vi "DronePi Main.vi"() -> ()   [LabVIEW 2014]
uses:
  SubVI/Aircraft Information/Controls/Drone Information.ctl
  SubVI/Aircraft Information/Controls/Base Mode.ctl
  SubVI/Aircraft Information/Controls/Aircraft Mode.ctl
  SubVI/Aircraft Information/Controls/Aircraft Sensor Status Data.ctl
  SubVI/GUI Design/Indicators/Sensor Status LED CLuster.ctl
  SubVI/GUI Design/Indicators/Status LED.ctl
  SubVI/Aircraft Information/Controls/Aircraft GPS Data.ctl
  SubVI/Aircraft Information/Controls/GPS Fix Type.ctl
  SubVI/Aircraft Information/Controls/Aircraft Attitude Data.ctl
  <vilib>/Platform/TimedLoop/XDataNode/timing_clust.ctl
  <vilib>/Platform/TimedLoop/XDataNode/nitl_modes.ctl
  <vilib>/Platform/TimedLoop/XDataNode/wakeup.ctl
  SubVI/Aircraft Information/Sub VI/Selected Aircraft/SubVI/Set Selected Aircraft.vi
  Web Services/DronePi Global Variables.vi
  SubVI/Aircraft Information/Sub VI/Selected Aircraft/SubVI/Get Selected Aircraft.vi
  SubVI/Aircraft Information/Sub VI/Get Aircraft Attitude.vi
  SubVI/Aircraft Information/Sub VI/Get Aircraft GPS.vi
  SubVI/Aircraft Information/Sub VI/Get Aircraft System Status.vi
  SubVI/Aircraft Information/Sub VI/Get Aircraft Information.vi
  <vilib>/platform/TimedLoop/XDataNode/XDataNode.xnode
  <vilib>/Platform/TimedLoop/XDataNode/XDNodeRunTimeDep.lvlib
panel:
  out "Aircraft Att Data Out":T1
  out "Aircraft GPS Data Out":T2
  out "System Status Out":T4 {"Communication Drop Rate (%)" scale=0.0..100.0; "Battery Remaining (%)" scale=0.0..100.0; "CPU Load (%)" scale=0.0..100.0}
  out "Aircraft Information Out":T7={"Aircraft ID"=0, "Tag ID"="", "System Status"="", "Base Mode"={"Custom Mode"=FALSE, "Test Enabled"=FALSE, "Autonomous Mode"=FALSE, "Guided Mode"=FALSE, "Stabilization Enabled"=FALSE, "HIL Enabled"=FALSE, "Manual Mode"=FALSE, "Arm"=FALSE}, "Armed/Disarmed"=FALSE, "Battery Voltage"=0.0, "Control Mode"=enum."Stabalise", "Initialisation"=0, "Coms with aircraft good"=FALSE, "Mode"="", "Mission Uploaded"=FALSE} {"Initialisation" scale=0.0..100.0}
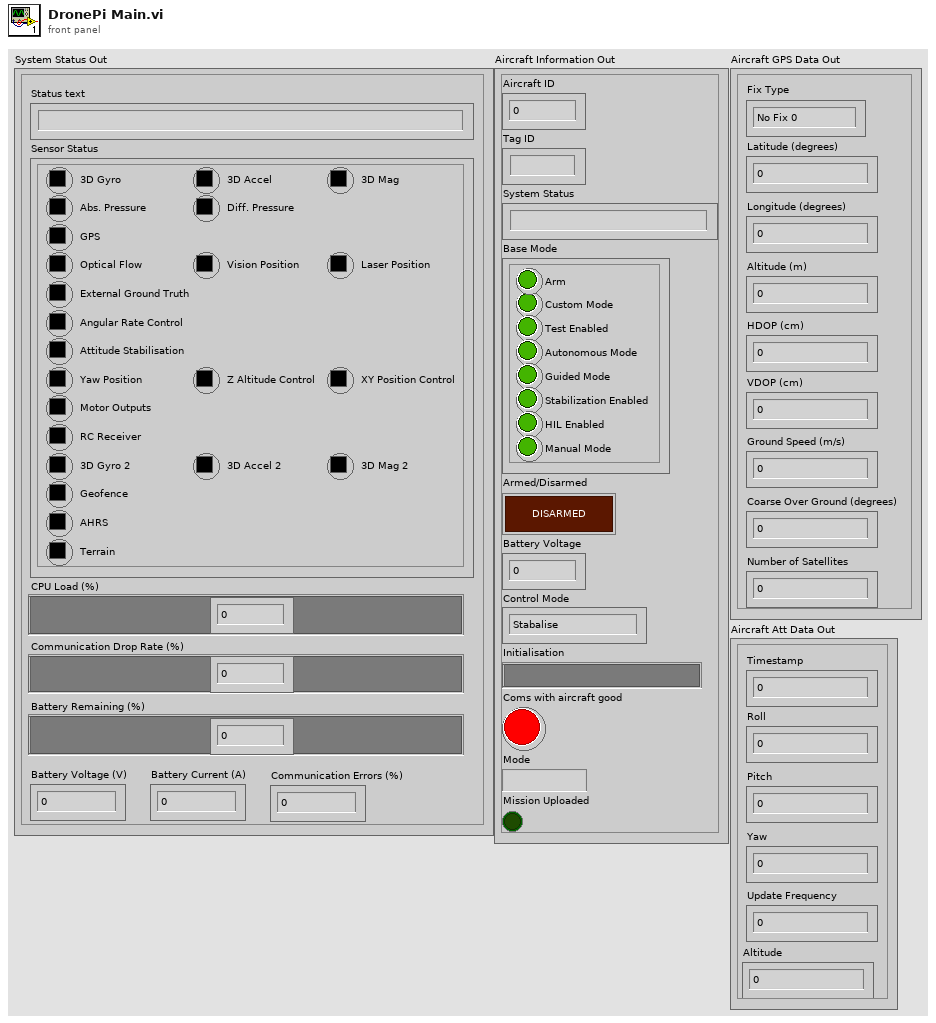
[diagram p1: front panel]
types:
  T1 = typedef "Aircraft Attitude Data.ctl" = cluster{"Roll":sgl, "Pitch":sgl, "Yaw":sgl, "Timestamp":u32, "Update Frequency":dbl, "Altitude":sgl}
  T2 = typedef "Aircraft GPS Data.ctl" = cluster{"Latitude (degrees)":dbl, "Longitude (degrees)":dbl, "Altitude (m)":dbl, "Fix Type":T3, "HDOP (cm)":u16, "VDOP (cm)":u16, "Ground Speed (m/s)":dbl, "Coarse Over Ground (degrees)":u16, "Number of Satellites":u8}
  T3 = typedef "GPS Fix Type.ctl" = enum16{"No Fix 0", "No Fix 1", "2D Fix", "3D Fix", "DGPS", "RTK"}
  T4 = typedef "Aircraft Sensor Status Data.ctl" = cluster{"Sensor Status":T5, "CPU Load (%)":dbl, "Battery Voltage (V)":dbl, "Battery Current (A)":dbl, "Battery Remaining (%)":dbl, "Communication Drop Rate (%)":dbl, "Communication Errors (%)":dbl, "Status text":string}
  T5 = typedef "Sensor Status LED CLuster.ctl" = cluster{"3D Gyro":u32, "3D Accel":u32, "3D Mag":u32, "Abs. Pressure":u32, "Diff. Pressure":u32, "GPS":T6, "Optical Flow":u32, "Vision Position":u32, "Laser Position":u32, "External Ground Truth":u32, "Angular Rate Control":u32, "Attitude Stabilisation":u32, "Yaw Position":u32, "Z Altitude Control":u32, "XY Position Control":u32, "Motor Outputs":u32, "RC Receiver":u32, "3D Gyro 2":u32, "3D Accel 2":u32, "3D Mag 2":u32, "Geofence":u32, "AHRS":u32, "Terrain":u32}
  T6 = typedef "Status LED.ctl" = u32
  T7 = typedef "Drone Information.ctl" = cluster{"Aircraft ID":u8, "Tag ID":string, "System Status":string, "Base Mode":T8, "Armed/Disarmed":bool, "Battery Voltage":dbl, "Control Mode":T9, "Initialisation":u8, "Coms with aircraft good":bool, "Mode":string, "Mission Uploaded":bool}
  T8 = typedef "Base Mode.ctl" = cluster{"Custom Mode":bool, "Test Enabled":bool, "Autonomous Mode":bool, "Guided Mode":bool, "Stabilization Enabled":bool, "HIL Enabled":bool, "Manual Mode":bool, "Arm":bool}
  T9 = typedef "Aircraft Mode.ctl" = enum16{"Loiter", "Stabalise", "Failsafe", "Emergency Stop"}
  T10 = typedef "XDNodeRunTimeDep.lvlib/timing_clust.ctl" = cluster{"Expected End [f-1]":u64, "Actual End [f-1]":u64, "Finished Late? [f-1]":bool, "Expected End [i-1]":u64, "Actual End [i-1]":u64, "Finished Late? [i-1]":bool, "Expected Start [i]":u64, "Actual Start [i]":u64, "Expected Start [f]":u64, "Actual Start [f]":u64, "Source Name":string, "Structure Name":string, "Period":i64, "Deadline":i64, "Offset":i64, "Start":i64, "Priority":i32, "Timeout":i32, "Mode":T11, "Wakeup Reason":T12, "Error":errorcluster, "Source Type":string, "Secondary Source Type":string, "Global End Time":u64, "Global Start Time":u64, "Frame Duration":u64, "Iteration Duration":u64, "Assigned CPU":i32, "I/O Scan Engine Mode":u32}
  T11 = typedef "XDNodeRunTimeDep.lvlib/nitl_modes.ctl" = enum32{"No Change", "Process missed periods, maintain original phase", "Discard missed periods, maintain original phase", "Process missed periods, ignore original phase", "Discard missed periods, ignore original phase"}
  T12 = typedef "XDNodeRunTimeDep.lvlib/wakeup.ctl" = enum32{"Normal", "Aborted", "Asynchronous wakeup", "Timing source error", "Timed loop error", "Timeout"}
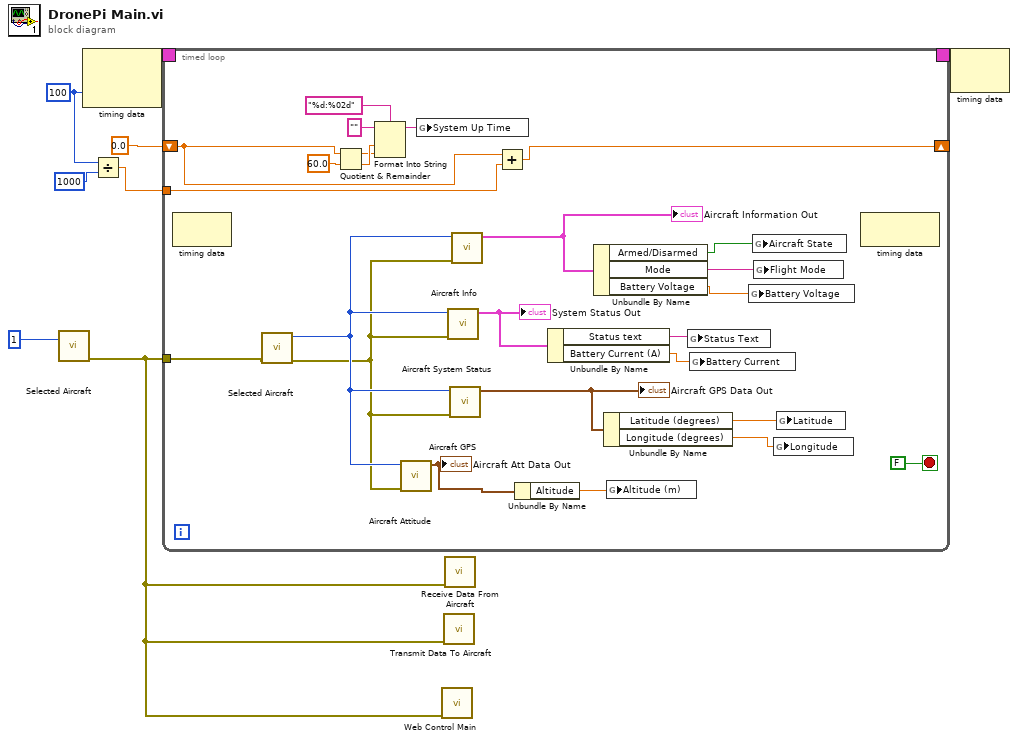
[diagram p0: block diagram]
diagram:
  w3 = i64 100 ("Period")
  n1 = call-poly "Selected Aircraft.vi"("Selected Aircraft ID In"=u8 1) -> ("Error Out"=w5:errorcluster)  [unwired: 10 in]
  n2 = node-c288(w3) -> (w8:T10)  [unwired: 1 in]
  n3 = Divide(x=w3, y=i64 1000) -> (x/y=w1:dbl)
  n4 = timed-loop {
    timing: w8 -> [_]
    timing-out: [_] -> w7
    tunnel: w5 -> [w30]
    shift-right: [w10] -> _
    shift-left: 0.0 ("relative seconds") -> [w9]
    tunnel: w1 -> [w11]
    stop <- FALSE stop-if-true
    n5 = node-c288() -> ()  [unwired: 1 in, 1 out]
    n6 = call-poly "Selected Aircraft.vi"("Error In"=w30) -> ("Error Out"=w24:errorcluster, "Selected Aircraft ID Out"=w25:u8)  [unwired: 9 in]
    n7 = Quotient & Remainder(x=w9, y=60.0) -> (x-y*floor(x/y)=w15:dbl, floor(x/y)=w16:dbl)
    n8 = Format Into String(format string="%d:%02d", initial string="", w16, w15) -> (resulting string=w12:string)  [unwired: 1 in, 1 out]
    n9 = call-poly "Aircraft Attitude.vi"("Error In"=w24, "Aircraft ID"=w25) -> ("Aircraft Att Data Out"=w23:T1)  [unwired: 8 in, 1 out]
    "Aircraft Att Data Out" <- w23
    n10 = global write "DronePi Global Variables.vi" "System Up Time"(w12) -> ()
    n11 = call-poly "Aircraft System Status.vi"("Error In"=w24, "Aircraft ID"=w25) -> ("System Status Out"=w21:T4)  [unwired: 8 in, 1 out]
    "System Status Out" <- w21
    n12 = call-poly "Aircraft GPS.vi"("Error In"=w24, "Aircraft ID"=w25) -> ("Aircraft GPS Data Out"=w28:T2)  [unwired: 8 in, 1 out]
    "Aircraft GPS Data Out" <- w28
    n13 = call-poly "Aircraft Info.vi"("Error In"=w24, "Aircraft ID"=w25) -> ("Aircraft Information Out"=w32:T7)  [unwired: 8 in, 1 out]
    "Aircraft Information Out" <- w32
    n14 = Add(x=w9, y=w11) -> (x+y=w10:dbl)
    n15 = Unbundle By Name(w23) -> ("Altitude"=w22:sgl)
    n16 = Unbundle By Name(w21) -> ("Status text"=w20:string, "Battery Current (A)"=w19:dbl)
    n17 = Unbundle By Name(w32) -> ("Armed/Disarmed"=w18:bool, "Mode"=w31:string, "Battery Voltage"=w29:dbl)
    n18 = Unbundle By Name(w28) -> ("Latitude (degrees)"=w27:dbl, "Longitude (degrees)"=w26:dbl)
    n19 = global write "DronePi Global Variables.vi" "Altitude (m)"(w22) -> ()
    n20 = global write "DronePi Global Variables.vi" "Status Text"(w20) -> ()
    n21 = global write "DronePi Global Variables.vi" "Battery Current"(w19) -> ()
    n22 = global write "DronePi Global Variables.vi" "Battery Voltage"(w29) -> ()
    n23 = global write "DronePi Global Variables.vi" "Aircraft State"(w18) -> ()
    n24 = global write "DronePi Global Variables.vi" "Flight Mode"(w31) -> ()
    n25 = global write "DronePi Global Variables.vi" "Longitude"(w26) -> ()
    n26 = global write "DronePi Global Variables.vi" "Latitude"(w27) -> ()
    n27 = node-c288() -> ()  [unwired: 1 in, 1 out]
  }
  n28 = call "Web Control Main.vi"("Error In"=w5) -> ()  [unwired: 10 in, 1 out]
  n29 = call "Transmit Data To Aircraft.vi"("Error In"=w5) -> ()  [unwired: 11 in]
  n30 = call "Receive Data From Aircraft.vi"("error in (no error)"=w5) -> ()  [unwired: 10 in, 1 out]
  n31 = node-c288(w7) -> ()  [unwired: 1 out]
